vi "main.vi"() -> ()   [LabVIEW 2017]
panel:
  out "output cluster":cluster{dbl, dbl}
  out "XY Graph":cluster{"X":dbl, "Y":dbl}[](graph)
  in  "Numer punktu":i32
  in  "Rysuj punkt":bool
  in  "Usuñ ostatni punkt":bool
  in  "Usuñ punkt o numerze":bool
  in  "Koniec":bool
  in  "Y":dbl(slide) scale=0.0..10.0
  in  "X":dbl(slide) scale=0.0..10.0
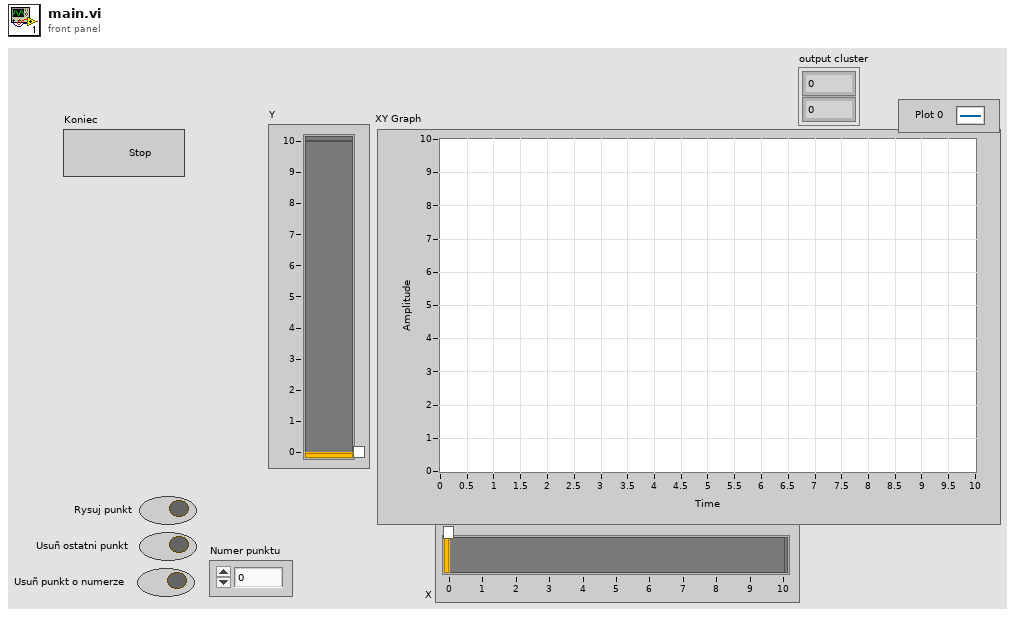
[diagram p1: front panel]
types:
  T1 = typedef "LVPoint32TypeDef.ctl" = cluster{"Horizontal":i32, "Vertical":i32}
  T2 = typedef "LVRectTypeDef.ctl" = cluster{"Left":i16, "Top":i16, "Right":i16, "Bottom":i16}
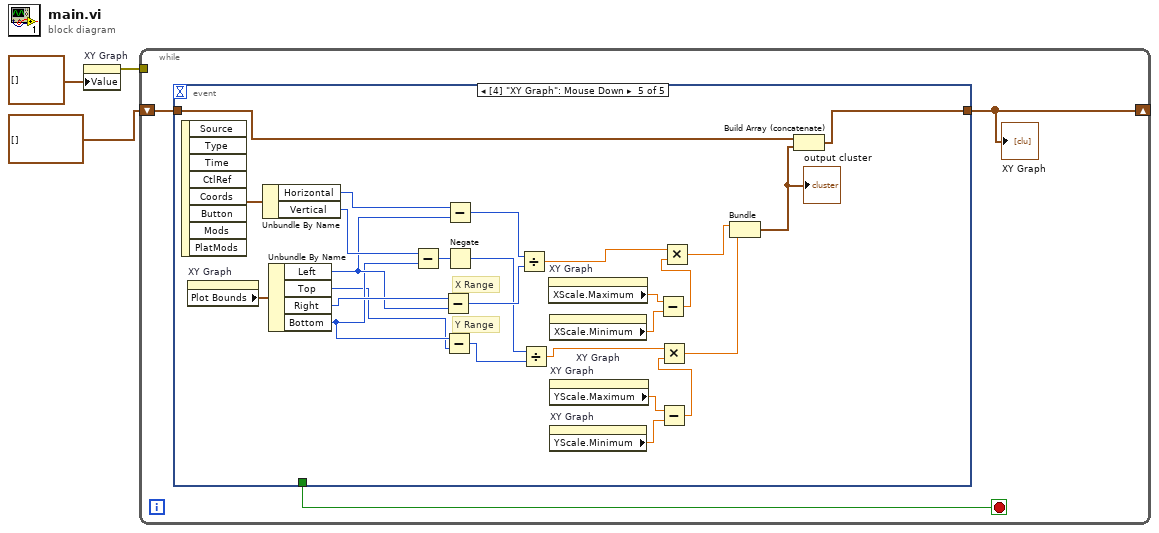
[diagram p0: block diagram]
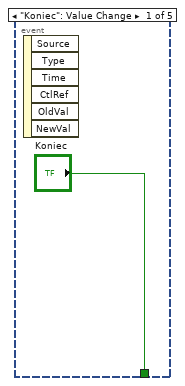
[diagram p2: hidden frame]
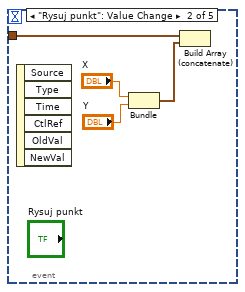
[diagram p3: hidden frame]
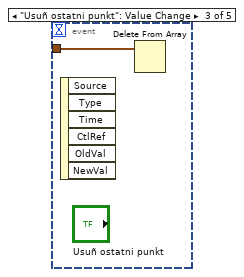
[diagram p4: hidden frame]
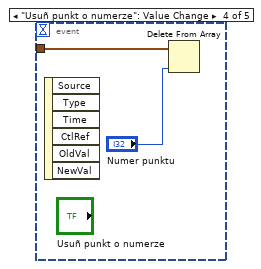
[diagram p5: hidden frame]
diagram:
  n1 = property on="XY Graph" class="XYGraph (strict)"("Value"=cluster{"X":dbl, "Y":dbl}[] [] ("XY Graph")) -> (error out=w1:errorcluster)  [unwired: 2 in, 1 out]
  n2 = while {
    shift-right: [w4] -> _
    shift-left: cluster{"X":dbl, "Y":dbl}[] [] ("XY Graph") -> [w5]
    tunnel: w1 -> [_]
    stop <- w6 stop-if-true
    n3 = event shown="[4] \"XY Graph\": Mouse Down" {
      selector: _ -> [_ _ _ _ _]
      dyn-events: _ -> [_ _ _ _ _]
      timeout: _ -> [_ _ _ _ _]
      tunnel: ["Koniec" _ _ _ _] -> w6
      tunnel: w5 -> [_ w9 w12 w14 w40]
      tunnel: [_ _ _ _ w39] -> w4
      event "Koniec": Value Change {
        n4 = event-data() -> ()  [unwired: 1 in, 6 out]
      }
      event "Rysuj punkt": Value Change {
        n5 = event-data() -> ()  [unwired: 1 in, 6 out]
        n6 = Bundle("X"="X", "Y"="Y") -> (w8:cluster{"X":dbl, "Y":dbl})  [unwired: 1 in]
        n7 = Build Array (concatenate)(w9, w8) -> ()  [unwired: 1 out]
      }
      event "Usuñ ostatni punkt": Value Change {
        n8 = event-data() -> ()  [unwired: 1 in, 6 out]
        n9 = Delete From Array(array=w12) -> ()  [unwired: 2 in, 2 out]
      }
      event "Usuñ punkt o numerze": Value Change {
        n10 = event-data() -> ()  [unwired: 1 in, 6 out]
        n11 = Delete From Array(array=w14, index="Numer punktu") -> ()  [unwired: 1 in, 2 out]
      }
      event "XY Graph": Mouse Down {
        # "Y Range"
        # "X Range"
        n12 = event-data() -> ("Coords"=w38:T1)  [unwired: 1 in, 7 out]
        n13 = property on="XY Graph" class="XYGraph (strict)"() -> ("Plot Bounds"=w37:T2)  [unwired: 2 in, 2 out]
        n14 = Unbundle By Name(w38) -> ("Horizontal"=w36:i32, "Vertical"=w35:i32)
        n15 = Unbundle By Name(w37) -> ("Left"=w32:i16, "Top"=w25:i16, "Right"=w33:i16, "Bottom"=w26:i16)
        n16 = Subtract(x=w35, y=w26) -> (x-y=w34:i32)
        n17 = Subtract(x=w33, y=w32) -> (x-y=w30:i16)
        n18 = Subtract(x=w26, y=w25) -> (x-y=w23:i16)
        n19 = Subtract(x=w36, y=w32) -> (x-y=w31:i32)
        n20 = Negate(x=w34) -> (-x=w24:i32)
        n21 = Divide(x=w31, y=w30) -> (x/y=w29:dbl)
        n22 = Divide(x=w24, y=w23) -> (x/y=w22:dbl)
        n23 = property on="XY Graph" class="XYGraph (strict)"() -> ("XScale.Maximum"=w17:dbl)  [unwired: 2 in, 2 out]
        n24 = property on="XY Graph" class="XYGraph (strict)"() -> ("XScale.Minimum"=w16:dbl)  [unwired: 2 in, 2 out]
        n25 = property on="XY Graph" class="XYGraph (strict)"() -> ("YScale.Maximum"=w20:dbl)  [unwired: 2 in, 2 out]
        n26 = property on="XY Graph" class="XYGraph (strict)"() -> ("YScale.Minimum"=w19:dbl)  [unwired: 2 in, 2 out]
        n27 = Subtract(x=w17, y=w16) -> (x-y=w15:dbl)
        n28 = Subtract(x=w20, y=w19) -> (x-y=w18:dbl)
        n29 = Multiply(x=w22, y=w18) -> (x*y=w21:dbl)
        n30 = Multiply(x=w29, y=w15) -> (x*y=w28:dbl)
        n31 = Bundle(w28, w21) -> (w27:cluster{dbl, dbl})  [unwired: 1 in]
        "output cluster" <- w27
        n32 = Build Array (concatenate)(w40, w27) -> (w39:cluster{"X":dbl, "Y":dbl}[])
      }
    }
    "XY Graph" <- w4
  }
